vi "Read Page Menu Properties.vi"(8 "Error In":errorcluster, 11 "Custom Device Page .NET Ref In":refnum<k24>) -> (0 "Error Out":errorcluster, 2 "All Menu Properties":T1[](array[typedef]), 3 "Custom Device Page .NET Ref Out":refnum<k24>)   [LabVIEW 2015, in "VeriStand Custom Device XML Parser.lvlib"]
doc: "Reads and returns the properties of all menus of the page"
uses:
  VeriStand Custom Device XML Parser.lvlib
  XML Controls/RuntTimeMenu Properties.ctl
  XML Controls/Execution Types.ctl
  XML Controls/Path Cluster.ctl
  XML Controls/Dependency Properties.ctl
  NationalInstruments.VeriStand.XMLReader
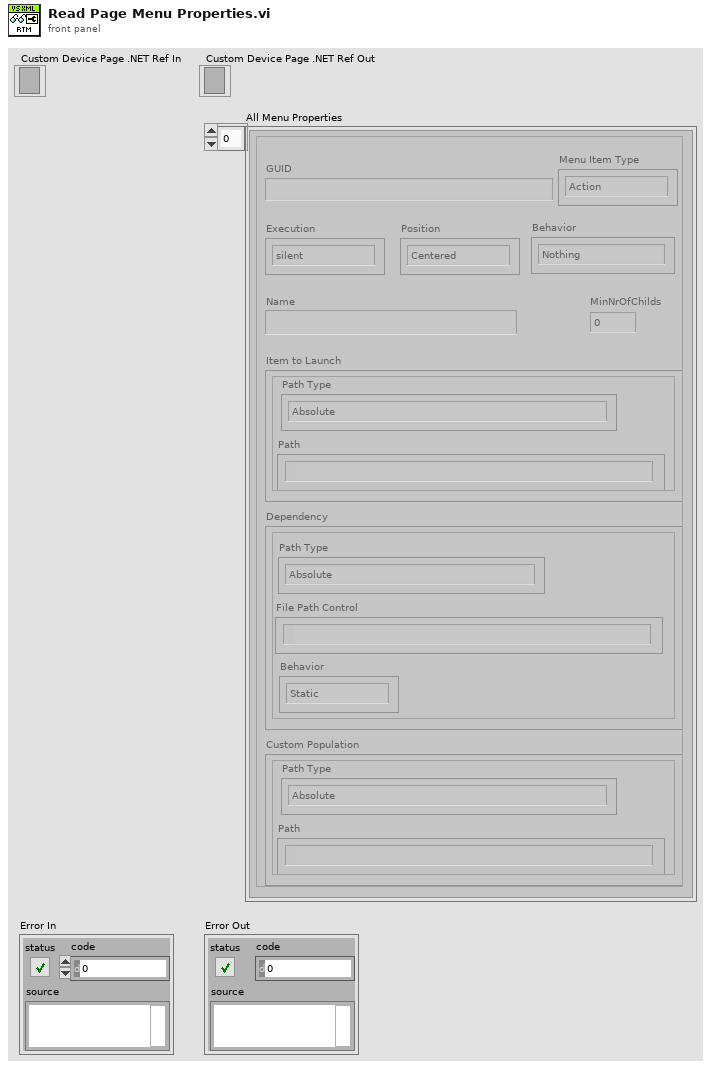
[diagram p1: front panel]
types:
  T1 = typedef "VeriStand Custom Device XML Parser.lvlib/RuntTimeMenu Properties.ctl" = cluster{"GUID":string, "Execution":T2, "MinNrOfChilds":u32, "Name":string, "Item to Launch":T3, "Dependency":T4, "Custom Population":T3, "Menu Item Type":enum16{"Action", "VI", "Separator", "Custom"}, "Behavior":enum16{"Nothing", "Open Front Panel"}, "Position":enum16{"Centered", "Mouse Pointer"}}
  T2 = typedef "VeriStand Custom Device XML Parser.lvlib/Execution Types.ctl" = enum16{"silent", "modal", "floating", "default"}
  T3 = typedef "VeriStand Custom Device XML Parser.lvlib/Path Cluster.ctl" = cluster{"Path":path, "Path Type":enum16{"Absolute", "To Base", "To Common Doc Dir", "To Application Data Dir"}}
  T4 = typedef "VeriStand Custom Device XML Parser.lvlib/Dependency Properties.ctl" = cluster{"File Path Control":path, "Path Type":enum16{"Absolute", "To Base", "To Common Doc Dir", "To Application Data Dir"}, "Behavior":enum16{"Static", "Dynamic"}}
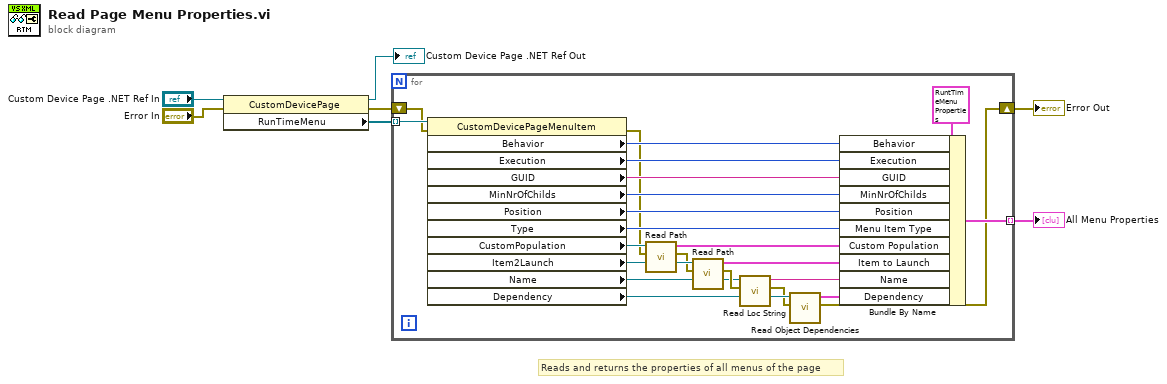
[diagram p0: block diagram]
diagram:
  # "Reads and returns the properties of all menus of the page"
  n1 = property class="CustomDevicePage"(reference="Custom Device Page .NET Ref In", error in="Error In") -> (reference out=→"Custom Device Page .NET Ref Out":refnum<k24>, error out=w4:errorcluster, "RunTimeMenu"=w3:refnum<k24>[])
  n2 = for {
    tunnel: w3 -> [w29] mode=indexing
    shift-right: [w8] -> w7
    shift-left: w4 -> [w28]
    tunnel: [w12] -> w6 mode=indexing
    n3 = property class="CustomDevicePageMenuItem"(reference=w29, error in=w28) -> (error out=w20:errorcluster, "Behavior"=w27:i32, "Execution"=w26:i32, "GUID"=w25:string, "MinNrOfChilds"=w24:i32, "Position"=w23:i32, "Type"=w22:i32, "CustomPopulation"=w21:refnum<k24>, "Item2Launch"=w19:refnum<k24>, "Name"=w14:refnum<k24>, "Dependency"=w11:refnum<k24>)  [unwired: 1 out]
    n4 = call "Read Path.vi"("Error In"=w20, "Path .NET Ref"=w21) -> ("Error Out"=w18:errorcluster, "Path Properties"=w17:T3)  [unwired: 8 in]
    n5 = call "Read Path.vi"("Error In"=w18, "Path .NET Ref"=w19) -> ("Error Out"=w15:errorcluster, "Path Properties"=w16:T3)  [unwired: 8 in]
    n6 = call "Read Loc String.vi"("Error In"=w15, "Loc String .NET Ref"=w14) -> ("Error Out"=w10:errorcluster, "English"=w13:string)  [unwired: 7 in, 1 out]
    n7 = call "Read Object Dependencies.vi"("Error In"=w10, "Dependency .NET Ref In"=w11) -> ("Error Out"=w8:errorcluster, "Dependency Properties"=w9:T4)  [unwired: 8 in]
    n8 = Bundle By Name(cluster=T1 {"GUID"="", "Execution"=enum."silent", "MinNrOfChilds"=0, "Name"="", "Item to Launch"={"Path"=path "", "Path Type"=enum."Absolute"}, "Dependency"={"File Path Control"=path "", "Path Type"=enum."Absolute", "Behavior"=enum."Static"}, "Custom Population"={"Path"=path "", "Path Type"=enum."Absolute"}, "Menu Item Type"=enum."Action", "Behavior"=enum."Nothing", "Position"=enum."Centered"} ("Menu Item"), "Behavior"=w27, "Execution"=w26, "GUID"=w25, "MinNrOfChilds"=w24, "Position"=w23, "Menu Item Type"=w22, "Custom Population"=w17, "Item to Launch"=w16, "Name"=w13, "Dependency"=w9) -> (w12:T1)
  }
  "Error Out" <- w7
  "All Menu Properties" <- w6
